vi "Scan SN for Solder.vi"(8 "error in (no error)":errorcluster, 11 "VISA resource name":refnum<visa-resource-name>) -> (0 "error out":errorcluster, 3 "Barcode":string)   [LabVIEW 2019]
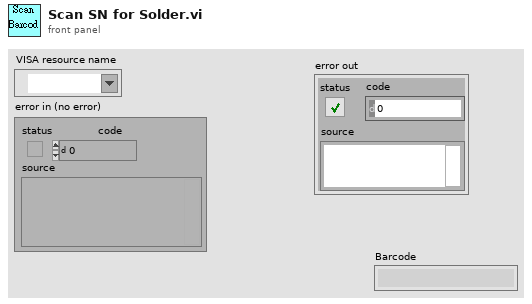
[diagram p1: front panel]
types:
  T1 = enum16{"Open", "Send", "Recieve", "Recieve cmd", "Close"}
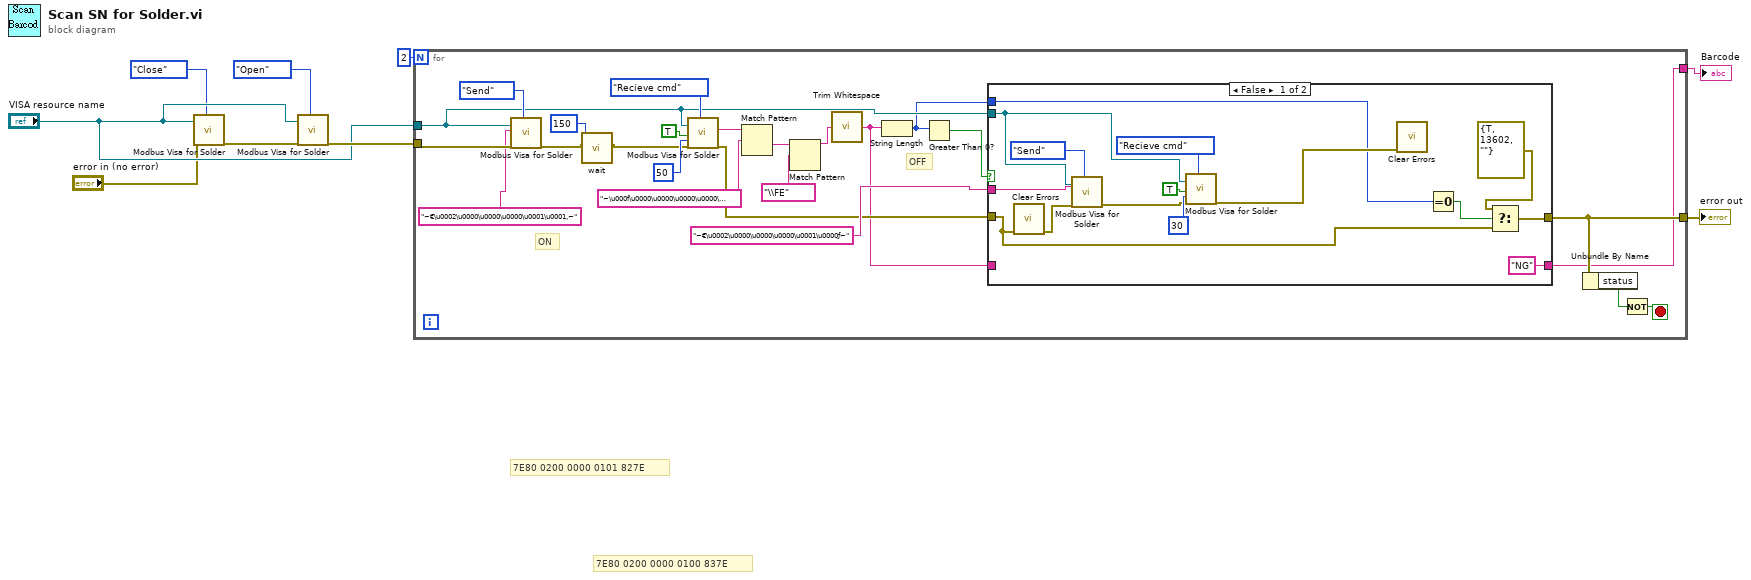
[diagram p0: block diagram]
diagram:
  # "7E80 0200 0000 0100 837E"
  # "7E80 0200 0000 0101 827E"
  n1 = call "Modbus Visa for Solder.vi"("VISA resource name"="VISA resource name", "error in (no error)"="error in (no error)", "VisaAction"=T1."Close") -> ("error out"=w4:errorcluster)  [unwired: 15 in, 1 out]
  n2 = call "Modbus Visa for Solder.vi"("VISA resource name"="VISA resource name", "error in (no error)"=w4, "VisaAction"=T1."Open") -> ("error out"=w8:errorcluster)  [unwired: 15 in, 1 out]
  n3 = for {
    N: 2 -> [_]
    tunnel: w8 -> [w33]
    tunnel: "VISA resource name" -> [w24]
    tunnel: [w29] -> w6
    tunnel: [w13] -> w1
    stop <- w30 stop-if-true
    # "OFF"
    # "ON"
    n4 = call "Modbus Visa for Solder.vi"("VISA resource name"=w24, "Cmd"="~€\u0002\u0000\u0000\u0000\u0001\u0001‚~", "error in (no error)"=w33, "VisaAction"=T1."Send") -> ("error out"=w11:errorcluster)  [unwired: 14 in, 1 out]
    n5 = call "wait.vi"("error in"=w11, "wait(ms)"=u32 150) -> ("error out"=w10:errorcluster)  [unwired: 9 in]
    n6 = call "Modbus Visa for Solder.vi"("VISA resource name"=w24, "TimeOut"=TRUE, "Time(0.1)"=u32 50, "error in (no error)"=w10, "VisaAction"=T1."Recieve cmd") -> ("read string"=w19:string, "error out"=w21:errorcluster)  [unwired: 13 in]
    n7 = Match Pattern(string=w19, regular expression="~\u000f\u0000\u0000\u0000\u0000\u0000\u000f~" ("trimmed string")) -> (after substring=w18:string)  [unwired: 1 in, 3 out]
    n8 = Match Pattern(string=w18, regular expression="\\FE") -> (before substring=w17:string)  [unwired: 1 in, 3 out]
    n9 = call <vilib>:"Trim Whitespace.vi"("string"=w17) -> ("trimmed string"=w14:string)  [unwired: 1 in]
    n10 = String Length(string=w14) -> (length=w15:i32)
    n11 = Greater Than 0?(x=w15) -> (x > 0?=w32:bool)
    n12 = case shown="False" w32 {
      tunnel: w21 -> [w45 w50]
      tunnel: [w44 w50] -> w29
      tunnel: w24 -> [w38 _]
      tunnel: "~€\u0002\u0000\u0000\u0000\u0001\u0000ƒ~" ("Cmd") -> [w37 _]
      tunnel: w15 -> [w35 _]
      tunnel: w14 -> [_ w49]
      tunnel: ["NG" ("trimmed string") w49] -> w13
      frame False {
        n13 = call <vilib>:"Clear Errors.vi"("error in (no error)"=w45) -> ("error out"=w48:errorcluster)  [unwired: 5 in, 1 out]
        n14 = call "Modbus Visa for Solder.vi"("VISA resource name"=w38, "Cmd"=w37, "error in (no error)"=w48, "VisaAction"=T1."Send") -> ("error out"=w39:errorcluster)  [unwired: 14 in, 1 out]
        n15 = call "Modbus Visa for Solder.vi"("VISA resource name"=w38, "TimeOut"=TRUE, "Time(0.1)"=u32 30, "error in (no error)"=w39, "VisaAction"=T1."Recieve cmd") -> ("error out"=w36:errorcluster)  [unwired: 13 in, 1 out]
        n16 = call <vilib>:"Clear Errors.vi"("error in (no error)"=w36) -> ()  [unwired: 5 in, 2 out]
        n17 = Equal To 0?(x=w35) -> (x = 0?=w46:bool)
        n18 = Select(t=errorcluster {"status"=TRUE, "code"=13602, "source"=""} ("error constant"), s=w46, f=w45) -> (s? t:f=w44:errorcluster)
      }
      frame True {
      }
    }
    n19 = Unbundle By Name(w29) -> ("status"=w31:bool)
    n20 = Not(x=w31) -> (.not. x?=w30:bool)
  }
  "error out" <- w6
  "Barcode" <- w1
